vi "VFH-read_folder-Excel.vi"() -> ()   [LabVIEW 2020]
uses:
  VFH-file_cluster-Expensive.ctl
  VFH-VNA_File_Handler.lvlib
panel:
  out "Array 2":dbl[](array[numeric])
  out "Array":T1[](array[typedef])
  in  "Folder Path":path
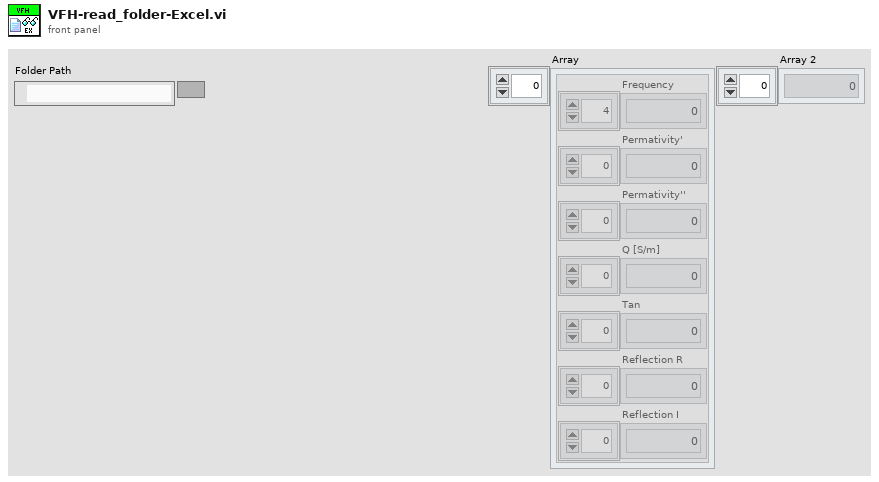
[diagram p1: front panel]
types:
  T1 = typedef "VFH-VNA_File_Handler.lvlib/VFH-file_cluster-Expensive.ctl" = cluster{"Frequency":dbl[], "Permativity'":dbl[], "Permativity''":dbl[], "Q [S/m]":dbl[], "Tan":dbl[], "Reflection R":dbl[], "Reflection I":dbl[]}
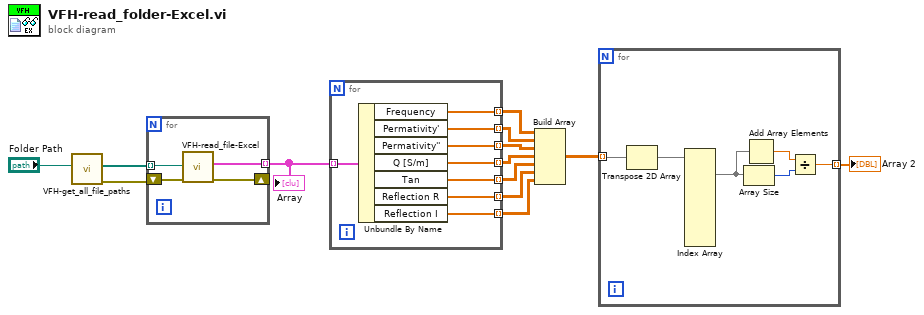
[diagram p0: block diagram]
diagram:
  n1 = call "VFH-get_all_file_paths.vi"("Folder Path"="Folder Path") -> ("error out"=w12:errorcluster, "All Files in Dir"=w11:path[])  [unwired: 8 in, 1 out]
  n2 = for {
    shift-right: [w15] -> _
    shift-left: w12 -> [w16]
    tunnel: w11 -> [w17] mode=indexing
    tunnel: [w14] -> w10 mode=indexing
    n3 = call "VFH-read_file-Excel.vi"("error in (no error)"=w16, "file path (dialog if empty)"=w17) -> ("error out"=w15:errorcluster, "output cluster"=w14:T1)  [unwired: 8 in]
  }
  "Array" <- w10
  n4 = for {
    tunnel: w10 -> [w25] mode=indexing
    tunnel: [w24] -> w9 mode=indexing
    tunnel: [w23] -> w8 mode=indexing
    tunnel: [w22] -> w7 mode=indexing
    tunnel: [w21] -> w6 mode=indexing
    tunnel: [w20] -> w5 mode=indexing
    tunnel: [w19] -> w4 mode=indexing
    tunnel: [w18] -> w3 mode=indexing
    n5 = Unbundle By Name(w25) -> ("Frequency"=w24:dbl[], "Permativity'"=w23:dbl[], "Permativity''"=w22:dbl[], "Q [S/m]"=w21:dbl[], "Tan"=w20:dbl[], "Reflection R"=w19:dbl[], "Reflection I"=w18:dbl[])
  }
  n6 = Build Array(w9, w8, w7, w6, w5, w4, w3) -> (w2:dbl[][][])
  n7 = for {
    tunnel: w2 -> [w31] mode=indexing
    tunnel: [w26] -> w1 mode=indexing
    n8 = Transpose 2D Array(2D array=w31) -> (transposed array=w30:dbl[][])
    n9 = Index Array(array=w30) -> (element #1=w29:dbl[])  [unwired: 10 in, 4 out]
    n10 = Array Size(array=w29) -> (size(s)=w27:i32)
    n11 = Add Array Elements(numeric array=w29) -> (sum=w28:dbl)
    n12 = Divide(x=w28, y=w27) -> (x/y=w26:dbl)
  }
  "Array 2" <- w1
